vi "Read Ports.vi"(0 "Refnum in":refnum<k20>, 2 "timeout (ms)":i32=5000, 5 "All 4 Ports":bool, 9 "number of elements":u64, 11 "error in":errorcluster, 13 "Simulated Data":bool) -> (4 "Refnum out":refnum<k20>, 6 "Receive Waveform":u64[](array[numeric]), 8 "Errors":u32[](array[numeric]), 10 "Elements Remaining":u32, 14 "Data Valid":bool, 15 "error out":errorcluster)   [LabVIEW 2016, in "Aurora Stream (NI 6592R) (Host).lvlib"]
doc: "This VI wraps and calls the appropriate FIFO read node to access the FIFO corresponding to the input <b>port</b>\n\n<B>Input Parameters</B>\n\n<B>Refnum in</B> Receives a reference to the FPGA from the previous VI.\n\n<B>timeout (ms)</B> The timeout to pass to the FIFO read node\n\n<B>port</B> Selects which physical port to read from.\n\n<B>number of elements</B> Specifies the number of FIFO elements to read during this call.\n\n<B>error in</B> describes error conditions that occur before this node runs. This input provides standard error in functionality.\n\n<B>Output Parameters</B>\n\n<B>Refnum out</B> passes a reference to the FPGA to the next VI.\n\n<B>Receive Waveform</B> The data read from the device will be written to this output\n\n<B>Waveform Size</B> Indicates the number of samples in the output waveform\n\n<B>Elements Remaining</B> Indicates the number of samples presently waiting in the FIFO after the read.\n\n<B>error out</B> contains error information. This output provides standard error out functionality."
uses:
  Aurora Stream (NI 6592R) (Host).lvlib
  Base Bitfile Reference.ctl
  <vilib>/Utility/error.llb/Error Cluster From Error Code.vi
  <vilib>/rvi/errors/niLvFpgaAdjustHostInterfaceError.vi
  <vilib>/rvi/interface/nirviMethod/nirviMethod.xnode
  <vilib>/rvi/interface/nirviReadWriteControl/nirviReadWriteControl.xnode
  <vilib>/FPGAPlugInAG/Dynamic/niLvFpga_ReadFifo_Dynamic.vi
  <vilib>/rvi/errors/niLvFpgaMergeErrorWithErrorCode.vi
  NiFpgaLv.dll
  <vilib>/rvi/interface/Simulation/niFpgaSimulationCallBeginRW.vi
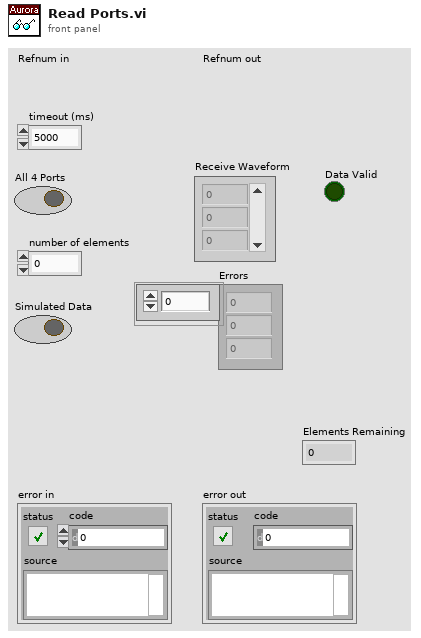
[diagram p1: front panel]
types:
  T1 = typedef "Aurora Stream (NI 6592R) (Host).lvlib/Base Bitfile Reference.ctl" = refnum<k20>
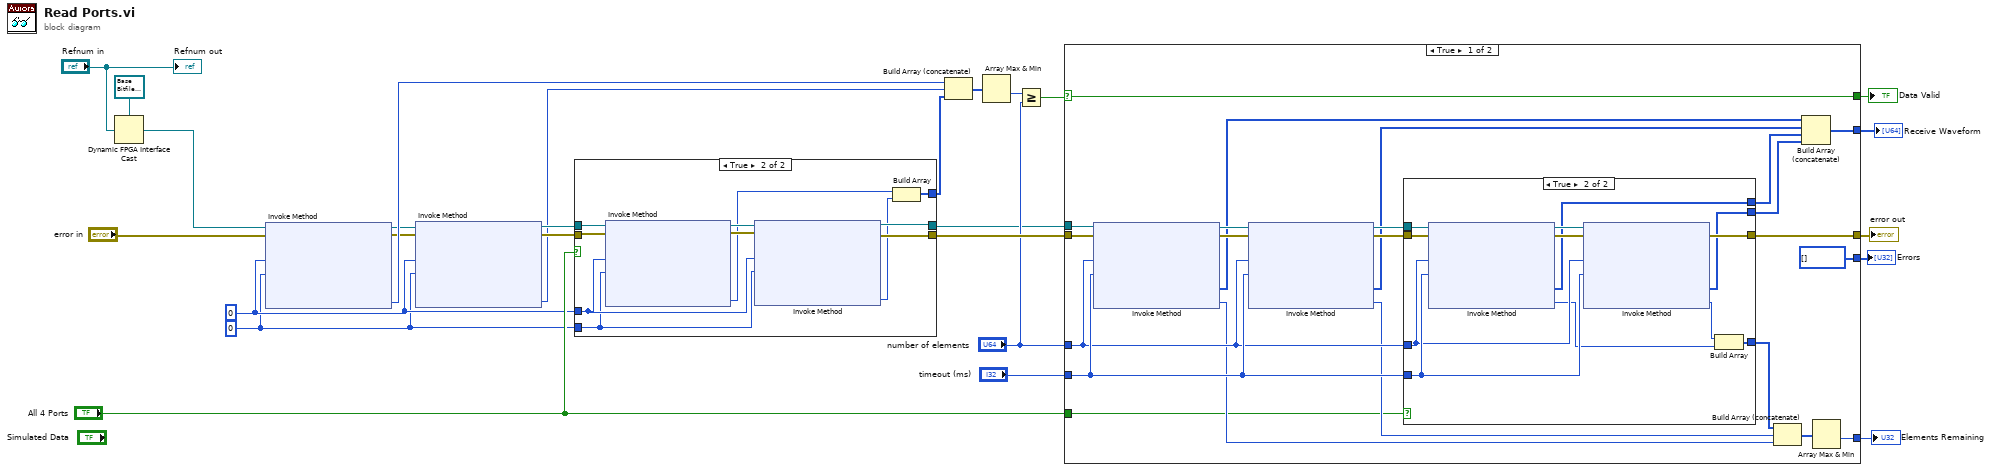
[diagram p0: block diagram]
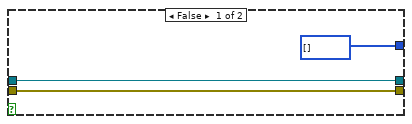
[diagram p2: hidden frame]
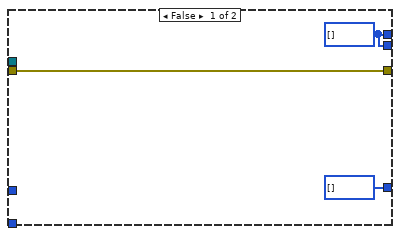
[diagram p3: hidden frame]
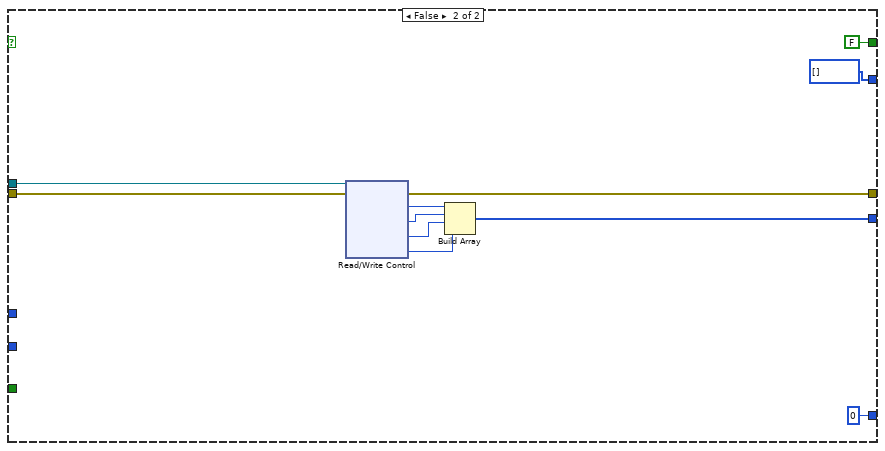
[diagram p4: hidden frame]
diagram:
  w2 = 0 ("Timeout (ms)")
  w3 = u32 0 ("Number of Elements")
  n1 = Dynamic FPGA Interface Cast(Session In=T1 refnum ("Aurora Sample Project"), Type="Refnum in") -> (Session Out=w12:T1)
  n2 = xnode "Invoke Method"("FPGA VI Reference In"=w12, "error in"="error in", "Number of Elements"=w3, "Timeout (ms)"=w2) -> ("FPGA VI Reference Out"=w9:T1, "error out"=w8:errorcluster, "Elements Remaining"=w10:u32)  [unwired: 1 out]
  n3 = xnode "Invoke Method"("FPGA VI Reference In"=w9, "error in"=w8, "Number of Elements"=w3, "Timeout (ms)"=w2) -> ("FPGA VI Reference Out"=w6:T1, "error out"=w7:errorcluster, "Elements Remaining"=w5:u32)  [unwired: 1 out]
  n4 = case shown="True" "All 4 Ports" {
    tunnel: w7 -> [w27 w38]
    tunnel: [w27 w35] -> w19
    tunnel: [u32[] [] w30] -> w22
    tunnel: w6 -> [w28 w37]
    tunnel: [w28 w36] -> w4
    tunnel: w3 -> [_ w34]
    tunnel: w2 -> [_ w33]
    frame False {
    }
    frame True {
      n5 = xnode "Invoke Method"("FPGA VI Reference In"=w37, "error in"=w38, "Number of Elements"=w34, "Timeout (ms)"=w33) -> ("FPGA VI Reference Out"=w39:T1, "error out"=w40:errorcluster, "Elements Remaining"=w32:u32)  [unwired: 1 out]
      n6 = xnode "Invoke Method"("FPGA VI Reference In"=w39, "error in"=w40, "Number of Elements"=w34, "Timeout (ms)"=w33) -> ("FPGA VI Reference Out"=w36:T1, "error out"=w35:errorcluster, "Elements Remaining"=w31:u32)  [unwired: 1 out]
      n7 = Build Array(w32, w31) -> (w30:u32[])
    }
  }
  n8 = Build Array (concatenate)(w10, w5, w22) -> (w21:u32[])
  n9 = Array Max & Min(array=w21) -> (min value=w20:u32)  [unwired: 3 out]
  n10 = Greater Or Equal?(x=w20, y="number of elements") -> (x >= y?=w18:bool)
  n11 = case shown="True" w18 {
    selector: w18 -> [w41 _]
    tunnel: [w55 w85] -> w26
    tunnel: "timeout (ms)" -> [w57 _]
    tunnel: w19 -> [w62 w86]
    tunnel: "number of elements" -> [w56 _]
    tunnel: "All 4 Ports" -> [w45 _]
    tunnel: [w50 u32 0] -> w15
    tunnel: [w42 u64[] []] -> w14
    tunnel: [u32[] [] w80] -> w13
    tunnel: w4 -> [w43 w79]
    tunnel: [w41 FALSE] -> w1
    frame True {
      n12 = xnode "Invoke Method"("FPGA VI Reference In"=w43, "error in"=w62, "Number of Elements"=w56, "Timeout (ms)"=w57) -> ("FPGA VI Reference Out"=w60:T1, "error out"=w61:errorcluster, "Data"=w49:u64[], "Elements Remaining"=w52:u32)
      n13 = xnode "Invoke Method"("FPGA VI Reference In"=w60, "error in"=w61, "Number of Elements"=w56, "Timeout (ms)"=w57) -> ("FPGA VI Reference Out"=w58:T1, "error out"=w59:errorcluster, "Data"=w48:u64[], "Elements Remaining"=w53:u32)
      n14 = case shown="True" w45 {
        tunnel: w59 -> [w65 w75]
        tunnel: w58 -> [_ w74]
        tunnel: w57 -> [_ w73]
        tunnel: w56 -> [_ w72]
        tunnel: [w65 w71] -> w55
        tunnel: [u32[] [] w68] -> w51
        tunnel: [w63 w67] -> w47
        tunnel: [w63 w66] -> w46
        frame False {
          w63 = u64[] [] ("Data")
        }
        frame True {
          n15 = xnode "Invoke Method"("FPGA VI Reference In"=w74, "error in"=w75, "Number of Elements"=w72, "Timeout (ms)"=w73) -> ("FPGA VI Reference Out"=w77:T1, "error out"=w76:errorcluster, "Data"=w67:u64[], "Elements Remaining"=w69:u32)
          n16 = xnode "Invoke Method"("FPGA VI Reference In"=w77, "error in"=w76, "Number of Elements"=w72, "Timeout (ms)"=w73) -> ("error out"=w71:errorcluster, "Data"=w66:u64[], "Elements Remaining"=w70:u32)  [unwired: 1 out]
          n17 = Build Array(w70, w69) -> (w68:u32[])
        }
      }
      n18 = Build Array (concatenate)(w51, w53, w52) -> (w54:u32[])
      n19 = Build Array (concatenate)(w49, w48, w47, w46) -> (w42:u64[])
      n20 = Array Max & Min(array=w54) -> (min value=w50:u32)  [unwired: 3 out]
    }
    frame False {
      n21 = xnode "Read/Write Control"("FPGA VI Reference In"=w79, "error in"=w86) -> ("error out"=w85:errorcluster, "Er.Port 0"=w84:u32, "Er.Port 1"=w83:u32, "Er.Port 2"=w82:u32, "Er.Port 3"=w81:u32)  [unwired: 1 out]
      n22 = Build Array(w84, w83, w82, w81) -> (w80:u32[])
    }
  }
  "Receive Waveform" <- w14
  "error out" <- w26
  "Elements Remaining" <- w15
  "Errors" <- w13
  "Data Valid" <- w1
  "Refnum out" <- "Refnum in"
